vi "Cal Inst - read electrical data.vi"(8 "error in (no error)":errorcluster, 11 "VISA Refnum in":refnum<visa-resource-name>) -> (0 "error out":errorcluster, 1 "Electrical Data":dbl[](array[numeric]), 2 "Electrical data labels":string[](array[string]), 3 "VISA Refnum out":refnum<visa-resource-name>)   [LabVIEW 2013]
uses:
  Libraries/California Instruments iX Series/California Instruments iX Series.lvlib
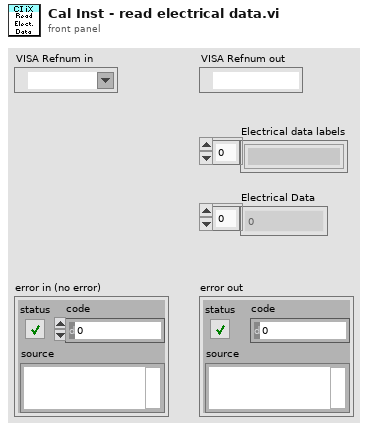
[diagram p1: front panel]
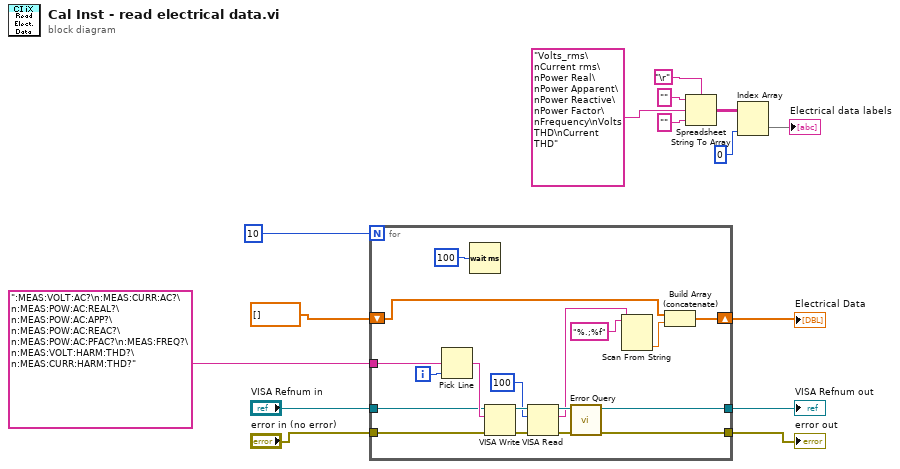
[diagram p0: block diagram]
diagram:
  n1 = for {
    N: 10 -> [_]
    tunnel: [w33] -> w4
    tunnel: [w32] -> w5
    tunnel: "VISA Refnum in" -> [w23]
    tunnel: "error in (no error)" -> [w22]
    shift-right: [w21] -> w7
    shift-left: dbl[] [] -> [w20]
    tunnel: ":MEAS:VOLT:AC?\n:MEAS:CURR:AC?\n:MEAS:POW:AC:REAL?\n:MEAS:POW:AC:APP?\n:MEAS:POW:AC:REAC?\n:MEAS:POW:AC:PFAC?\n:MEAS:FREQ?\n:MEAS:VOLT:HARM:THD?\n:MEAS:CURR:HARM:THD?" ("multi-line string") -> [w16]
    i -> [w18]
    n2 = Pick Line(multi-line string=w16, line index=w18) -> (output string=w24:string)  [unwired: 1 in]
    n3 = Wait (ms)(milliseconds to wait=u32 100) -> ()  [unwired: 1 out]
    n4 = VISA Write(VISA resource name=w23, write buffer=w24, error in (no error)=w22) -> (VISA resource name out=w31:refnum<visa-resource-name>, error out=w30:errorcluster)  [unwired: 1 out]
    n5 = VISA Read(VISA resource name=w31, byte count=u32 100, error in (no error)=w30) -> (VISA resource name out=w29:refnum<visa-resource-name>, read buffer=w26:string, error out=w28:errorcluster)  [unwired: 1 out]
    n6 = call "Error Query.vi"("error in (no error)"=w28, "VISA resource name"=w29) -> ("error out"=w33:errorcluster, "VISA resource name out"=w32:refnum<visa-resource-name>)  [unwired: 6 in, 2 out]
    n7 = Scan From String(format string="%.;%f", input string=w26) -> (output 1=w19:dbl)  [unwired: 3 in, 3 out]
    n8 = Build Array (concatenate)(w20, w19) -> (w21:dbl[])
  }
  "Electrical Data" <- w7
  "VISA Refnum out" <- w5
  "error out" <- w4
  n9 = Spreadsheet String To Array(delimiter (Tab)="\r", format string="", spreadsheet string="Volts_rms\nCurrent rms\nPower Real\nPower Apparent\nPower Reactive\nPower Factor\nFrequency\nVolts THD\nCurrent THD", array type (2D Dbl)="") -> (array=w14:string[][])
  n10 = Index Array(array=w14, index (col)=0) -> (element=→"Electrical data labels":string[])  [unwired: 1 in]
